vi "Copy Linked List.vi"(5 "Recursive? (T)":bool=TRUE, 6 "Insertion Index":i32=-1, 7 "New Parent Linked List ID":string, 8 "error in (no error)":errorcluster, 9 "New Linked List ID":string, 10 "Linked List ID":string, 11 "ILinked List in":refnum<class "ILinked List.lvclass">) -> (0 "error out":errorcluster, 2 "Linked List ID out":string, 3 "ILinked List out":refnum<class "ILinked List.lvclass">, 4 "Children":string[](array[string]))   [LabVIEW 2020, in "Linked Lists.lvlib" / "ILinked List.lvclass"]
uses:
  <vilib>/gpm_packages/@cs/linked-list/Source/Linked List/ILinkedList/ILinked List.lvclass
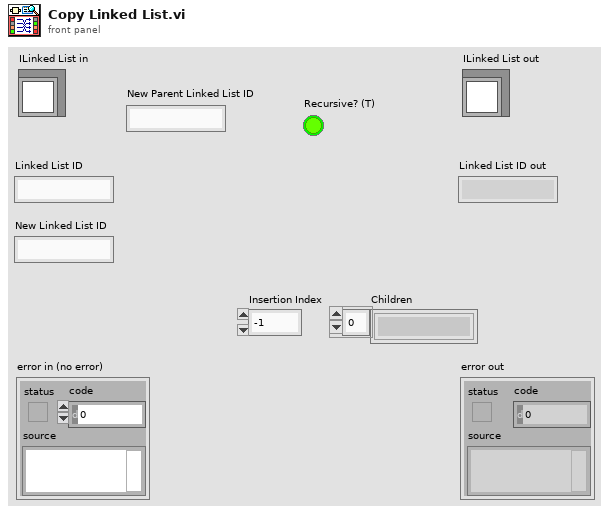
[diagram p1: front panel]
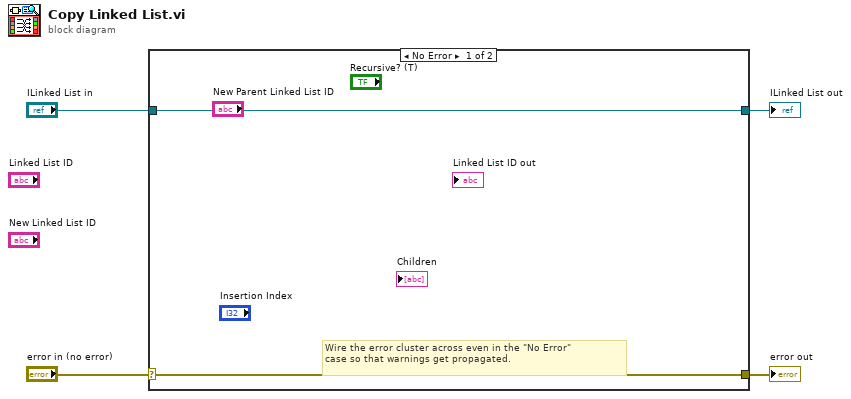
[diagram p0: block diagram]
diagram:
  n1 = case shown="No Error" "error in (no error)" {
    selector: "error in (no error)" -> [w5 w8]
    tunnel: [w5 w8] -> w3
    tunnel: [w6 w7] -> w1
    tunnel: "ILinked List in" -> [w6 w7]
    frame No Error {
      # "Wire the error cluster across even in the \"No Error\"\ncase so that warnings get propagated."
    }
    frame Error {
    }
  }
  "error out" <- w3
  "ILinked List out" <- w1
